vi "Aero_Chilled_Water_PID.vi"(1 "Tweak in working section demanded temp":dbl, 2 "Present Value":dbl=15.0 format="%.2f", 3 "Reset PID":bool, 4 "Setpoint":dbl=15.0 format="%.2f") -> (0 "Dem Output":dbl format="%.2f")   [LabVIEW 2010]
uses:
  <vilib>/Analysis/NI_AALPro.lvlib
panel:
  in  "O/P deadband":dbl=1.0 format="%.2f"
  in  "Kp Deadband":dbl format="%.2f"
  in  "Derivative History":i32=30
  out "deadbanded error":dbl format="%.2f"
  in  "P":bool=TRUE
  in  "D":bool=TRUE
  in  "I":bool=TRUE
  out "Waveform Chart":T1(graph)
  in  "Manual Demand":dbl min=0.0 max=100.0 format="%.2f"
  in  "Manual Override":bool
  out "Control Sum":dbl format="%.2f"
  out "Derivative Term":dbl format="%.2f"
  out "Integral Term":dbl format="%.2f"
  out "error differential":dbl format="%.5f"
  out "error integral":dbl format="%.2f"
  out "Proportional Term":dbl format="%.2f"
  in  "Kd":dbl=300.0 format="%.2f"
  in  "Ki":dbl=2.0 format="%.2f"
  in  "Kp":dbl=15.0 format="%.2f"
  out "error":dbl format="%.2f"
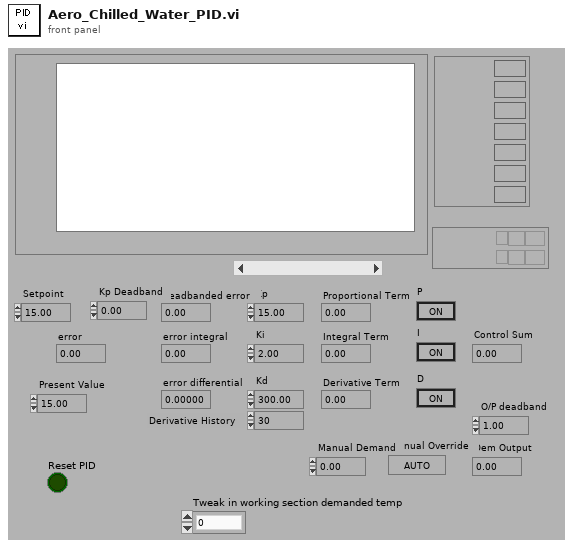
[diagram p1: front panel]
types:
  T1 = cluster{"Setpoint":dbl, "Present Value":dbl, "Proportional Term":dbl, "Integral Term":dbl, "Derivative Term":dbl, "Control Sum":dbl, "Dem Output":dbl}
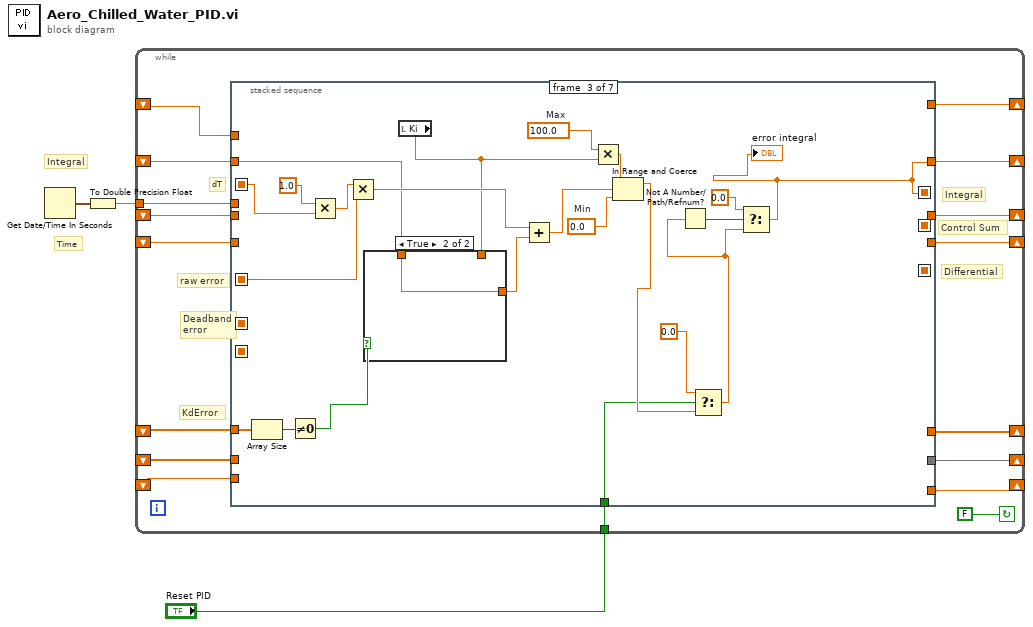
[diagram p0: block diagram]
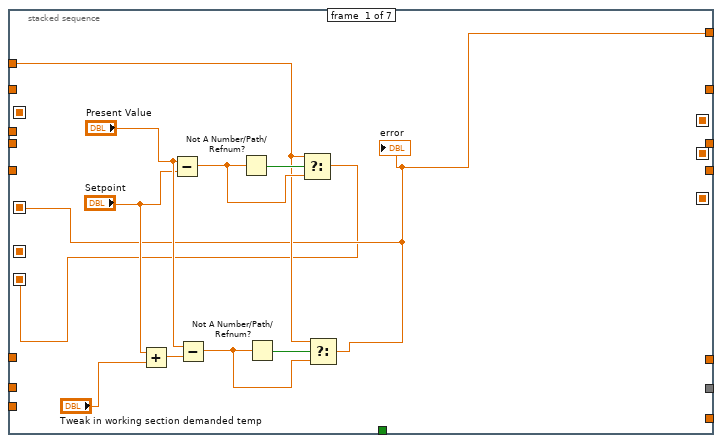
[diagram p2: hidden frame]
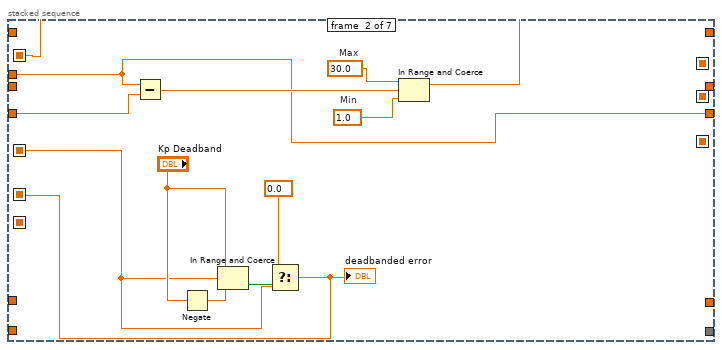
[diagram p3: hidden frame]
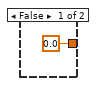
[diagram p4: hidden frame]
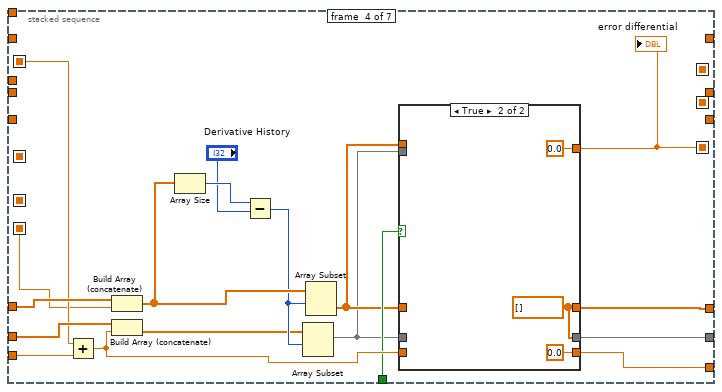
[diagram p5: hidden frame]
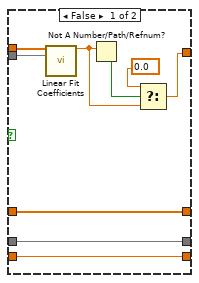
[diagram p6: hidden frame]
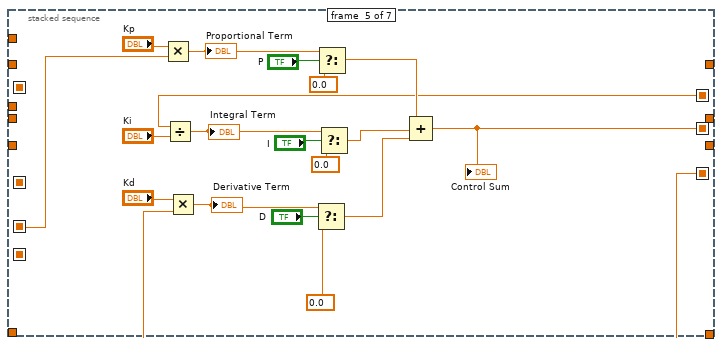
[diagram p7: hidden frame]
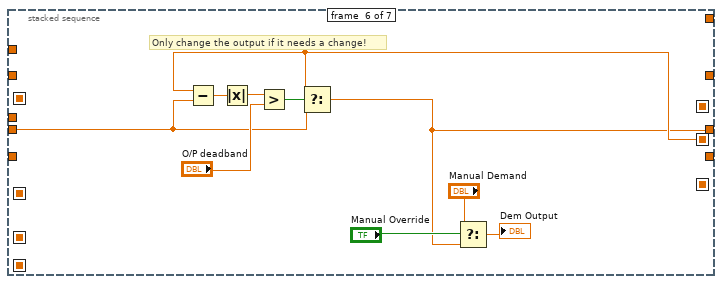
[diagram p8: hidden frame]
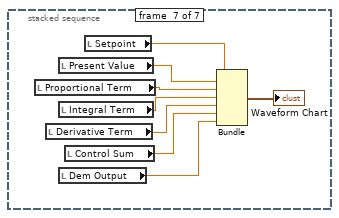
[diagram p9: hidden frame]
diagram:
  # "Integral"
  # "Time"
  n1 = Get Date/Time In Seconds() -> (seconds since 1Jan1904=w2:timestamp)
  n2 = To Double Precision Float(number=w2) -> (double precision float=w3:dbl)
  n3 = while {
    shift-left: _ -> [w7]
    shift-right: [w6] -> _
    shift-left: _ -> [w9]
    shift-right: [w8] -> _
    shift-left: _ -> [w11]
    shift-right: [w10] -> _
    tunnel: w3 -> [w16]
    shift-left: _ -> [w13]
    shift-right: [w12] -> _
    shift-left: _ -> [w15]
    shift-right: [w14] -> _
    shift-left: _ -> [w17]
    shift-right: [w18] -> _
    shift-left: _ -> [w20]
    shift-right: [w19] -> _
    tunnel: "Reset PID" -> [w4]
    stop <- FALSE continue-if-true
    # "KdError"
    # "Control Sum"
    # "raw error"
    # "Differential"
    # "Integral"
    # "Deadband\nerror"
    # "dT"
    n4 = stacked-sequence {
      seq-local: [_ w32 _ _ _ _ _] -> [_ _ w50 w77 _ _ _]
      seq-local: [_ w41 _ _ _ _ _] -> [_ _ _ _ w101 _ _]
      seq-local: [_ _ _ w78 _ _ _] -> [_ _ _ _ w100 _ _]
      seq-local: [_ _ w52 _ _ _ _] -> [_ _ _ _ w99 _ _]
      seq-local: [w22 _ _ _ _ _ _] -> [_ w33 w61 _ _ _ _]
      seq-local: [_ _ _ _ w104 _ _] -> [_ _ _ _ _ w120 _]
      seq-local: [w21 _ _ _ _ _ _] -> [_ _ _ w75 _ _ _]
      tunnel: w20 -> [_ w38 _ _ _ _ _]
      tunnel: [_ w36 _ _ _ _ _] -> w19
      tunnel: [_ _ w52 _ _ _ _] -> w18
      tunnel: w17 -> [_ _ w48 _ _ _ _]
      tunnel: w16 -> [_ w36 _ _ _ _ _]
      tunnel: w15 -> [_ _ w60 w85 _ _ _]
      tunnel: [_ _ _ w71 _ _ _] -> w14
      tunnel: w13 -> [_ _ _ w84 _ _ _]
      tunnel: [_ _ _ w69 _ _ _] -> w12
      tunnel: w11 -> [_ _ _ _ _ w118 _]
      tunnel: [_ _ _ _ _ w117 _] -> w10
      tunnel: w9 -> [_ _ _ w76 _ _ _]
      tunnel: [_ _ _ w74 _ _ _] -> w8
      tunnel: w7 -> [w27 _ _ _ _ _ _]
      tunnel: [w22 _ _ _ _ _ _] -> w6
      tunnel: w4 -> [_ _ w44 w72 _ _ _]
      frame #0 {
        n5 = Add(x="Setpoint", y="Tweak in working section demanded temp") -> (x+y=w23:dbl)
        n6 = Subtract(x="Present Value", y="Setpoint") -> (x-y=w30:dbl)
        n7 = Subtract(x="Present Value", y=w23) -> (x-y=w29:dbl)
        n8 = Not A Number/Path/Refnum?(number/path/refnum=w30) -> (NaN/Path/Refnum?=w31:bool)
        n9 = Not A Number/Path/Refnum?(number/path/refnum=w29) -> (NaN/Path/Refnum?=w28:bool)
        n10 = Select(t=w27, s=w31, f=w30) -> (s? t:f=w21:dbl)
        n11 = Select(t=w27, s=w28, f=w29) -> (s? t:f=w22:dbl)
        "error" <- w22
      }
      frame #1 {
        w39 = 1.0  # Min
        w40 = 30.0  # Max
        n12 = Subtract(x=w36, y=w38) -> (x-y=w37:dbl)
        n13 = Negate(x="Kp Deadband") -> (-x=w35:dbl)
        n14 = In Range and Coerce(upper limit="Kp Deadband", x=w33, lower limit=w35) -> (In Range?=w42:bool)  [unwired: 1 out]
        n15 = Select(t=0.0, s=w42, f=w33) -> (s? t:f=w41:dbl)
        "deadbanded error" <- w41
        n16 = In Range and Coerce(upper limit=w40, x=w37, lower limit=w39) -> (coerced(x)=w32:dbl)  [unwired: 1 out]
      }
      frame #2 {
        w65 = 0.0  # Min
        w64 = 100.0  # Max
        n17 = Array Size(array=w60) -> (size(s)=w59:i32)
        n18 = Not Equal To 0?(x=w59) -> (x != 0?=w57:bool)
        n19 = Multiply(x=1.0, y=w50) -> (x*y=w49:dbl)
        n20 = Multiply(x=w49, y=w61) -> (x*y=w58:dbl)
        n21 = local read "Ki"() -> (w55:dbl)
        n22 = case shown="True" w57 {
          tunnel: [0.0 ("Min") w67] -> w56
          tunnel: w48 -> [_ w67]
          tunnel: w55 -> [_ _]
          frame False {
          }
          frame True {
          }
        }
        n23 = Add(x=w58, y=w56) -> (x+y=w62:dbl)
        n24 = Multiply(x=w64, y=w55) -> (x*y=w63:dbl)
        n25 = In Range and Coerce(upper limit=w63, x=w62, lower limit=w65) -> (coerced(x)=w46:dbl)  [unwired: 1 out]
        n26 = Select(t=0.0, s=w44, f=w46) -> (s? t:f=w45:dbl)
        n27 = Not A Number/Path/Refnum?(number/path/refnum=w45) -> (NaN/Path/Refnum?=w53:bool)
        n28 = Select(t=0.0, s=w53, f=w45) -> (s? t:f=w52:dbl)
        "error integral" <- w52
      }
      frame #3 {
        n29 = Add(x=w77, y=w76) -> (x+y=w73:dbl)
        n30 = Build Array (concatenate)(w85, w75) -> (w81:dbl[])
        n31 = Build Array (concatenate)(w84, w73) -> (w79:dbl[])
        n32 = Array Size(array=w81) -> (size(s)=w83:i32)
        n33 = Subtract(x=w83, y="Derivative History") -> (x-y=w80:i32)
        n34 = Array Subset(array=w79, index=w80) -> (w68:dbl[])  [unwired: 1 in]
        n35 = Array Subset(array=w81, index=w80) -> (w70:dbl[])  [unwired: 1 in]
        n36 = case shown="True" w72 {
          tunnel: w70 -> [w94 _]
          tunnel: [w88 0.0 ("slope")] -> w78
          tunnel: w68 -> [w93 _]
          tunnel: [w89 0.0] -> w74
          tunnel: w73 -> [w89 _]
          tunnel: [w87 w96] -> w71
          tunnel: w70 -> [w87 _]
          tunnel: [w86 w96] -> w69
          tunnel: w68 -> [w86 _]
          frame False {
            n37 = call <vilib>:"Linear Fit Coefficients.vi"("Y"=w94, "X"=w93) -> ("slope"=w90:dbl)  [unwired: 3 in, 10 out]
            n38 = Not A Number/Path/Refnum?(number/path/refnum=w90) -> (NaN/Path/Refnum?=w92:bool)
            n39 = Select(t=0.0 ("f"), s=w92, f=w90) -> (s? t:f=w88:dbl)
          }
          frame True {
            w96 = dbl[] []
          }
        }
        "error differential" <- w78
      }
      frame #4 {
        n40 = Multiply(x="Kp", y=w101) -> (x*y=w114:dbl)
        "Proportional Term" <- w114
        n41 = Divide(x=w99, y="Ki") -> (x/y=w105:dbl)
        "Integral Term" <- w105
        n42 = Multiply(x="Kd", y=w100) -> (x*y=w106:dbl)
        "Derivative Term" <- w106
        n43 = Select(t=w106, s="D", f=0.0) -> (s? t:f=w108:dbl)
        n44 = Select(t=w114, s="P", f=0.0) -> (s? t:f=w115:dbl)
        n45 = Select(t=w105, s="I", f=0.0) -> (s? t:f=w107:dbl)
        n46 = Compound Arithmetic op=ADD(w115, w107, w108) -> (w104:dbl)
        "Control Sum" <- w104
      }
      frame #5 {
        # "Only change the output if it needs a change!"
        n47 = Subtract(x=w120, y=w118) -> (x-y=w123:dbl)
        n48 = Absolute Value(x=w123) -> (abs(x)=w122:dbl)
        n49 = Greater?(x=w122, y="O/P deadband") -> (0:w121:bool)
        n50 = Select(t=w120, s=w121, f=w118) -> (s? t:f=w117:dbl)
        n51 = Select(t="Manual Demand", s="Manual Override", f=w117) -> (s? t:f=→"Dem Output":dbl)
      }
      frame #6 {
        n52 = local read "Proportional Term"() -> (w130:dbl)
        n53 = local read "Derivative Term"() -> (w132:dbl)
        n54 = local read "Present Value"() -> (w129:dbl)
        n55 = local read "Integral Term"() -> (w131:dbl)
        n56 = local read "Dem Output"() -> (w134:dbl)
        n57 = local read "Control Sum"() -> (w133:dbl)
        n58 = local read "Setpoint"() -> (w128:dbl)
        n59 = Bundle("Setpoint"=w128, "Present Value"=w129, "Proportional Term"=w130, "Integral Term"=w131, "Derivative Term"=w132, "Control Sum"=w133, "Dem Output"=w134) -> (→"Waveform Chart":T1)  [unwired: 1 out]
      }
    }
  }
